vi "In Place Sanity.vi"(5 "Reversed?":bool, 7 "Steer In":dbl, 8 "Throttle In":dbl) -> (1 "Steer Out":dbl, 2 "Throttle Out":dbl)   [LabVIEW 2020]
uses:
  <vilib>/Analysis/coordinate.llb/Angle Units.ctl
  <vilib>/Analysis/coordinate.llb/Angle Range (Degree).ctl
  <vilib>/Analysis/coordinate.llb/Angle Rotation (scalar).vi
  <vilib>/Analysis/coordinate.llb/Wrap Angle (scalar).vi
  <vilib>/Analysis/NI_AAL_Angle.lvlib
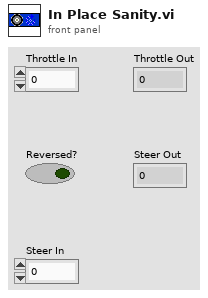
[diagram p1: front panel]
types:
  T1 = typedef "NI_AAL_Angle.lvlib/Angle Range (Degree).ctl" = u16
  T2 = typedef "NI_AAL_Angle.lvlib/Angle Units.ctl" = i32
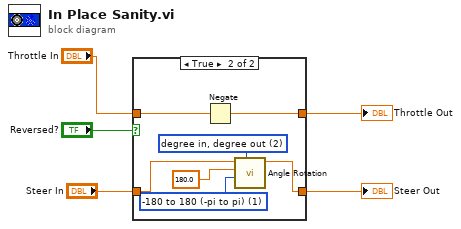
[diagram p0: block diagram]
diagram:
  n1 = case shown="True" "Reversed?" {
    tunnel: "Steer In" -> [w7 w12]
    tunnel: [w7 w10] -> w3
    tunnel: "Throttle In" -> [w6 w9]
    tunnel: [w6 w8] -> w4
    frame False {
    }
    frame True {
      w13 = T1 1 items=["none", "-180 to 180 (-pi to pi)", "0 to 360 (0 to 2pi)"] ("rotated angle range")
      w14 = T2 2 items=["radian in, radian out", "radian in, degree out", "degree in, degree out", "degree in, radian out"] ("angle units")
      n2 = Negate(x=w9) -> (-x=w8:dbl)
      n3 = call-poly <vilib>:"Angle Rotation.vi"("angle units"=w14, "rotated angle range"=w13, "counterclockwise rotation"=180.0, "angle"=w12) -> ("rotated angle"=w10:dbl)  [unwired: 6 in, 1 out]
    }
  }
  "Throttle Out" <- w4
  "Steer Out" <- w3
